vi "Get Counter Resource.vi"(0 "Task Name":refnum<k21>, 5 "channel":string) -> (4 "counter":tag)   [LabVIEW 2021, in "NIDAQmxMeasurement.lvlib"]
doc: "Gets the Counter resource from task name and channel name."
uses:
  NIDAQmxMeasurement.lvlib
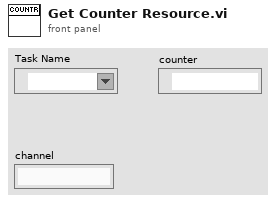
[diagram p1: front panel]
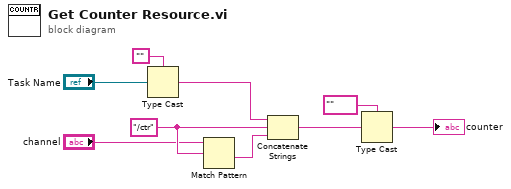
[diagram p0: block diagram]
diagram:
  w7 = "/ctr" ("regular expression")
  n1 = Type Cast(type="", x="Task Name") -> (*(type *) &x=w1:string)
  n2 = Match Pattern(string="channel", regular expression=w7) -> (after substring=w8:string)  [unwired: 1 in, 3 out]
  n3 = Concatenate Strings(w1, w7, w8) -> (w9:string)
  n4 = Type Cast(type=tag "" ("counter"), x=w9) -> (*(type *) &x=→"counter":tag)
